vi "RW_setparams_forloop.vi"(3 "error in (no error)":errorcluster caption="Error IN", 4 "Rotating Wall Parameters":T1={"Start Frequency"=9000.0, "Stop Frequency"=9000.0, "Sweep Time"=0.0, "Amplitude"=0.0, "Phase (ch.1)"=0.001, "Phase (Ch.2)"=90.0} {"Sweep Time" format="%.4f"; "Phase (Ch.2)" min=-1800.0 max=1800.0 step=0.1 format="%.3f"; "Phase (ch.1)" min=-1800.0 max=1800.0 step=0.1 format="%.3f"; "Stop Frequency" format="%#.5p"; "Start Frequency" format="%#.5p"; "Amplitude" min=0.0 max=4.0 format="%.3f"}, 5 "VISAsession":refnum<visa-resource-name>="wavefactoryU5") -> (0 "error out":errorcluster caption="Error OUT", 2 "CopyVISAsession":refnum<visa-resource-name>="wavefactoryU5")   [LabVIEW 2018]
panel:
  out "Elapsed Time":dbl=0.013423800000055053
  # "Have to manually set each wavefactory \nto 2-phase, sweep, 50 ohms (each channel)"
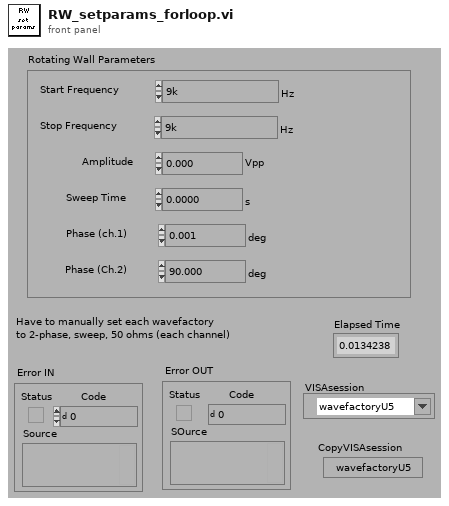
[diagram p1: front panel]
types:
  T1 = cluster{"Start Frequency":dbl, "Stop Frequency":dbl, "Sweep Time":dbl, "Amplitude":dbl, "Phase (ch.1)":dbl, "Phase (Ch.2)":dbl}
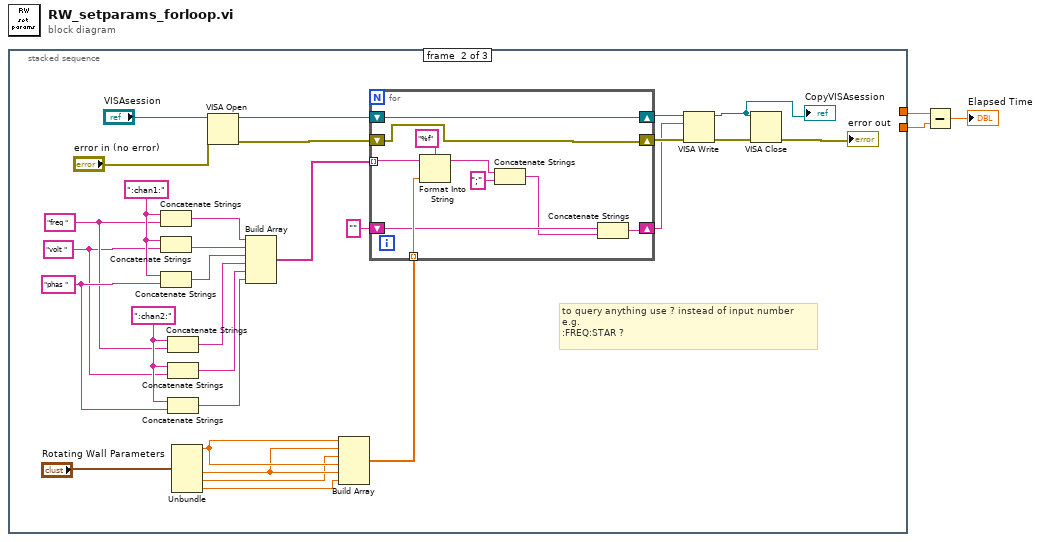
[diagram p0: block diagram]
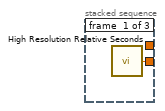
[diagram p2: hidden frame]
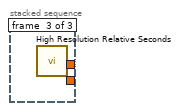
[diagram p3: hidden frame]
diagram:
  n1 = stacked-sequence {
    tunnel: [w4 _ _] -> w2
    tunnel: [_ _ w44] -> w3
    frame #0 {
      n2 = call <vilib>:"High Resolution Relative Seconds.vi"() -> ("relative seconds"=w4:dbl)
    }
    frame #1 {
      w18 = ":chan2:"
      w16 = "freq "
      w17 = "phas "
      w15 = "volt "
      w19 = ":chan1:"
      # "to query anything use ? instead of input number\ne.g.\n:FREQ:STAR ?"
      n3 = Concatenate Strings(w19, w16) -> (w14:string)
      n4 = Concatenate Strings(w19, w15) -> (w13:string)
      n5 = Concatenate Strings(w19, w17) -> (w12:string)
      n6 = Concatenate Strings(w18, w16) -> (w9:string)
      n7 = Concatenate Strings(w18, w15) -> (w10:string)
      n8 = Concatenate Strings(w18, w17) -> (w11:string)
      n9 = Unbundle("Rotating Wall Parameters") -> ("Start Frequency"=w8:dbl, "Amplitude"=w7:dbl, "Phase (ch.1)"=w5:dbl, "Phase (Ch.2)"=w6:dbl)  [unwired: 2 out]
      n10 = VISA Open(error in (no error)="error in (no error)", VISA resource name="VISAsession") -> (VISA resource name=w30:refnum<visa-resource-name>, error out=w29:errorcluster)  [unwired: 3 in]
      n11 = Build Array(w14, w13, w12, w9, w10, w11) -> (w20:string[])
      n12 = Build Array(w8, w7, w5, w8, w7, w6) -> (w22:dbl[])
      n13 = for {
        shift-right: [w37] -> w26
        shift-left: w30 -> [w37]
        shift-right: [w36] -> w25
        shift-left: w29 -> [w36]
        tunnel: w20 -> [w34] mode=indexing
        tunnel: w22 -> [w41] mode=indexing
        shift-right: [w40] -> w24
        shift-left: "" -> [w39]
        n14 = Format Into String(format string="%f", initial string=w34, w41) -> (resulting string=w42:string)  [unwired: 1 in, 1 out]
        n15 = Concatenate Strings(w42, ";" ("string")) -> (w38:string)
        n16 = Concatenate Strings(w39, w38) -> (w40:string)
      }
      n17 = VISA Write(VISA resource name=w26, write buffer=w24, error in (no error)=w25) -> (VISA resource name out=w27:refnum<visa-resource-name>, error out=w28:errorcluster)  [unwired: 1 out]
      "CopyVISAsession" <- w27
      n18 = VISA Close(VISA resource name=w27, error in (no error)=w28) -> (error out=→"error out":errorcluster)
    }
    frame #2 {
      n19 = call <vilib>:"High Resolution Relative Seconds.vi"() -> ("relative seconds"=w44:dbl)
    }
  }
  n20 = Subtract(x=w3, y=w2) -> (x-y=→"Elapsed Time":dbl)
